vi "Channel Selection Dialog.vi"(7 "DisplayFilter":u8(ring)=7 items=["K_CHAN_R", "K_CHAN_W", "K_CHAN_RW", "K_CHAN_VOLT", "K_CHAN_FAULT", "K_ALL", "K_CUSTOM", "K_CHAN_R_VIS", "K_CHAN_W_VIS", "K_CHAN_RW_VIS", "K_CHAN_VOLT_VIS", "K_CHAN_FAULT_VIS"], 8 "error in (no error)":errorcluster, 10 "Custom Data in":T1, 11 "NIVS.System Definition Root":refnum<k24>) -> (0 "error out":errorcluster, 1 "Cancelled":bool, 2 "Custom Data out":T1)   [LabVIEW 2014]
doc: "Use this template to create a dialog box with event handling."
uses:
  NationalInstruments.VeriStand.SystemStorageUI
  NationalInstruments.VeriStand.SystemStorage
  Boolean Control Timed Data.ctl
  NationalInstruments.VeriStand
  <vilib>/NI Veristand/UI Controls/Single Node Browser/NI_VS UI Single Node Browser.lvlib
panel:
  in  "Time (ms)":u32=100 min=100 step=100
  in  "Cancel":bool
  in  "Ok":bool
  in  "Selected Channel":refnum<k24>(container)
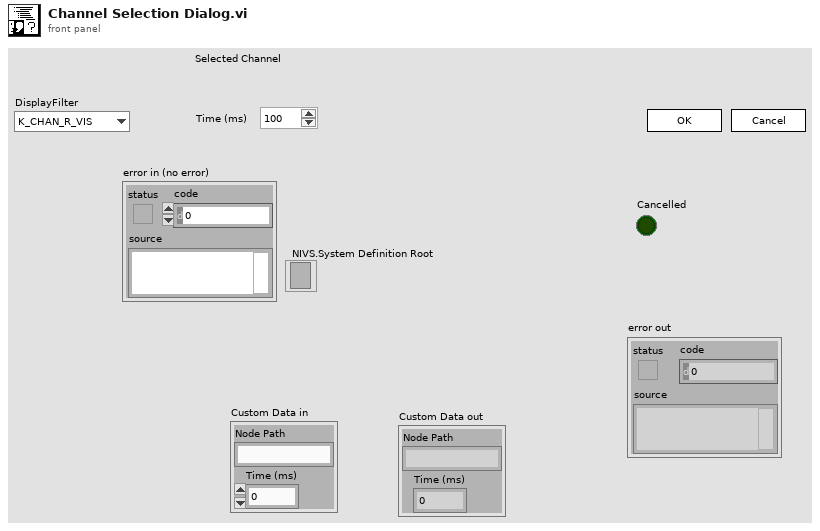
[diagram p1: front panel]
types:
  T1 = typedef "Boolean Control Timed Data.ctl" = cluster{"Node Path":string, "Time (ms)":u32}
  T2 = typedef "NI_VS UI Single Node Browser.lvlib/Callback Type.ctl" = cluster{"Net Callbacks":refnum<k27>[], "Event":refnum<user-event>}
  T3 = typedef "NI_VS UI Single Node Browser.lvlib/Node Ref.ctl" = refnum<k24>
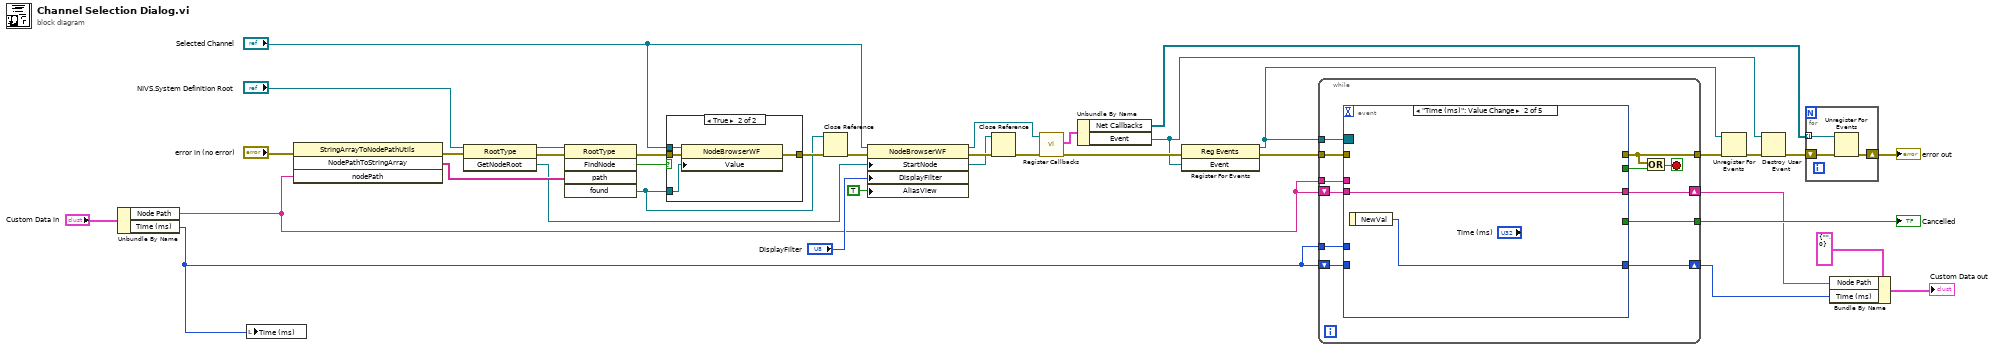
[diagram p0: block diagram]
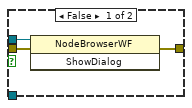
[diagram p2: hidden frame]
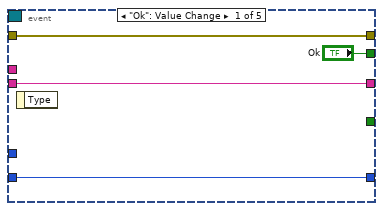
[diagram p3: hidden frame]
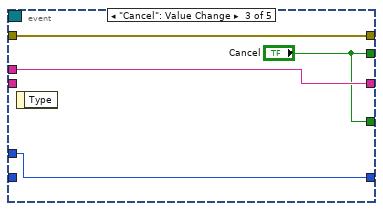
[diagram p4: hidden frame]
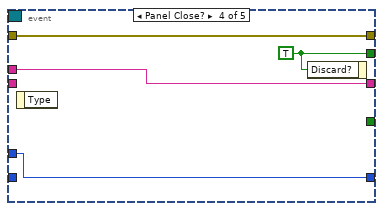
[diagram p5: hidden frame]
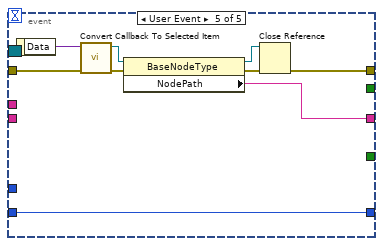
[diagram p6: hidden frame]
diagram:
  n1 = Unbundle By Name("Custom Data in") -> ("Node Path"=w6:string, "Time (ms)"=w5:u32)
  n2 = local write "Time (ms)"(w5) -> ()
  n3 = invoke class="StringArrayToNodePathUtils" method="NodePathToStringArray"(error in="error in (no error)", "nodePath"=w6) -> (error out=w15:errorcluster, "NodePathToStringArray"=w14:string[])  [unwired: 2 in, 2 out]
  n4 = invoke class="RootType" method="GetNodeRoot"(reference="NIVS.System Definition Root", error in=w15) -> (reference out=w34:refnum<k24>, error out=w35:errorcluster, "GetNodeRoot"=w9:refnum<k24>)  [unwired: 1 in]
  n5 = invoke class="RootType" method="FindNode"(reference=w34, error in=w35, "path"=w14) -> (error out=w28:errorcluster, "FindNode"=w27:bool, "found"=w11:refnum<k24>)  [unwired: 2 in, 2 out]
  n6 = case shown="True" w27 {
    tunnel: w11 -> [_ w41]
    tunnel: w28 -> [w39 w42]
    tunnel: [w37 w40] -> w25
    tunnel: "Selected Channel" -> [w38 w43]
    frame False {
      n7 = invoke class="NodeBrowserWF" method="ShowDialog"(reference=w38, error in=w39) -> (error out=w37:errorcluster)  [unwired: 1 in, 2 out]
    }
    frame True {
      n8 = property class="NodeBrowserWF"(reference=w43, error in=w42, "Value"=w41) -> (error out=w40:errorcluster)  [unwired: 1 out]
    }
  }
  n9 = Close Reference(reference=w11, error in (no error)=w25) -> (error out=w24:errorcluster)
  n10 = property class="NodeBrowserWF"(reference="Selected Channel", error in=w24, "StartNode"=w9, "DisplayFilter"="DisplayFilter", "AliasView"=TRUE) -> (reference out=w31:refnum<k24>, error out=w32:errorcluster)
  n11 = Close Reference(reference=w9, error in (no error)=w32) -> (error out=w10:errorcluster)
  n12 = call <vilib>:"Register Callbacks.vi"("error in (no error)"=w10, "Single Node Browser"=w31) -> ("error out"=w36:errorcluster, "Callbacks"=w33:T2)  [unwired: 7 in, 1 out]
  n13 = Unbundle By Name(w33) -> ("Net Callbacks"=w19:refnum<k27>[], "Event"=w18:refnum<user-event>)
  n14 = register-events(error in=w36, w18) -> (reference out=w21:refnum<event-registration>, error out=w26:errorcluster)  [unwired: 1 in]
  n15 = while {
    tunnel: [w48] -> w23
    tunnel: w26 -> [w54]
    tunnel: w21 -> [w52]
    shift-right: [w51] -> w3
    shift-left: w6 -> [w50]
    tunnel: w6 -> [w49]
    tunnel: [w47] -> w8
    tunnel: w5 -> [w46]
    shift-right: [w44] -> w2
    shift-left: w5 -> [w45]
    stop <- w53 stop-if-true
    n16 = event shown="[1] \"Time (ms)\": Value Change" {
      selector: w52 -> [_ _ _ _ _]
      dyn-events: _ -> [_ _ _ _ _]
      timeout: _ -> [_ _ _ _ _]
      tunnel: ["Ok" _ "Cancel" w69 _] -> w55
      tunnel: [w59 _ w65 w68 w76] -> w48
      tunnel: w54 -> [w59 _ w65 w68 w77]
      tunnel: [w57 w60 w64 w67 w71] -> w51
      tunnel: w50 -> [w57 w60 _ _ _]
      tunnel: w49 -> [_ _ w64 w67 _]
      tunnel: [_ _ "Cancel" _ _] -> w47
      tunnel: w46 -> [_ _ w62 w66 _]
      tunnel: w45 -> [w56 _ _ _ w70]
      tunnel: [w56 w61 w62 w66 w70] -> w44
      event "Ok": Value Change {
        n17 = event-data() -> ()  [unwired: 1 in, 1 out]
      }
      event "Time (ms)": Value Change {
        n18 = event-data() -> ("NewVal"=w61:u32)  [unwired: 1 in]
      }
      event "Cancel": Value Change {
        n19 = event-data() -> ()  [unwired: 1 in, 1 out]
      }
      event Panel Close? {
        w69 = TRUE ("Cancel")
        n20 = event-data() -> ()  [unwired: 1 in, 1 out]
        n21 = event-data("Discard?"=w69) -> ()  [unwired: 1 in, 1 out]
      }
      event User Event {
        n22 = event-data() -> ("Data"=w78:variant)  [unwired: 1 in]
        n23 = call <vilib>:"Convert Callback To Selected Item.vi"("error in"=w77, "Data"=w78) -> ("error out"=w72:errorcluster, "Selected Item"=w75:T3)  [unwired: 8 in]
        n24 = property class="BaseNodeType"(reference=w75, error in=w72) -> (reference out=w74:T3, error out=w73:errorcluster, "NodePath"=w71:string)
        n25 = Close Reference(reference=w74, error in (no error)=w73) -> (error out=w76:errorcluster)
      }
    }
    n26 = Or(x=w48, y=w55) -> (x .or. y?=w53:bool)
  }
  "Cancelled" <- w8
  n27 = Unregister For Events(event registration refnum=w21, error in=w23) -> (error out=w22:errorcluster)
  n28 = Destroy User Event(user event=w18, error in=w22) -> (error out=w20:errorcluster)
  n29 = for {
    tunnel: w19 -> [w80] mode=indexing
    shift-right: [w79] -> w13
    shift-left: w20 -> [w81]
    n30 = Unregister For Events(event registration refnum=w80, error in=w81) -> (error out=w79:errorcluster)
  }
  "error out" <- w13
  n31 = Bundle By Name(cluster=T1 {"Node Path"="", "Time (ms)"=0} ("Custom Data out"), "Node Path"=w3, "Time (ms)"=w2) -> (→"Custom Data out":T1)
